vi "Generate Hash Code.vi"(7 "Hash":enum16{"MD5", "FNV-1"}(ring)=enum."FNV-1", 10 "Fingerprint":string, 11 "Product ID":string) -> (2 "Hash":string, 3 "Encrypt":string)   [LabVIEW 2013]
uses:
  <userlib>/_OpenG.lib/md5/md5.llb/MD5 Message Digest (Hexadecimal String)__ogtk.vi
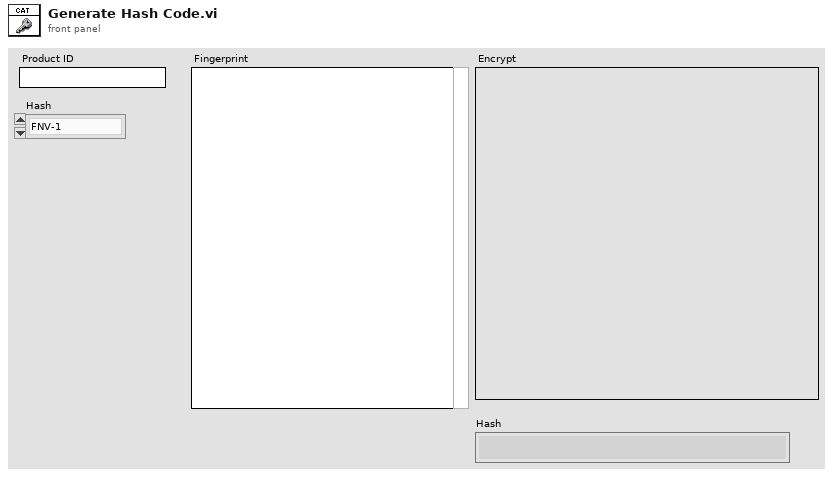
[diagram p1: front panel]
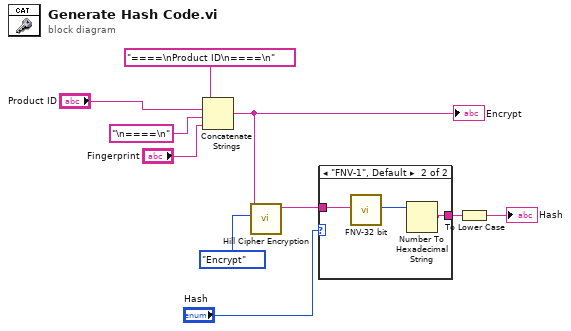
[diagram p0: block diagram]
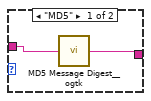
[diagram p2: hidden frame]
diagram:
  n1 = Concatenate Strings("====\nProduct ID\n====\n", "Product ID", "\n====\n" ("string"), "Fingerprint") -> (w10:string)
  "Encrypt" <- w10
  n2 = call <userlib>:"Hill Cipher Encryption.vi"("Operation"=enum16{"Encrypt", "Decrypt", "Decrypt from Hex"}."Encrypt", "Input String"=w10) -> ("Output String"=w4:string)  [unwired: 7 in, 2 out]
  n3 = case shown="\"FNV-1\", Default" "Hash" {
    tunnel: w4 -> [w12 w15]
    tunnel: [w11 w13] -> w2
    frame "MD5" {
      n4 = call-poly <userlib>:"MD5 Message Digest__ogtk.vi"("Message"=w12) -> ("MD5 Message Digest"=w11:string)
    }
    frame "FNV-1", Default {
      n5 = call "FNV-32 bit.vi"("Key"=w15) -> ("32 bit FNV-1 hash"=w14:u32)  [unwired: 18 in]
      n6 = Number To Hexadecimal String(2:w14) -> (0:w13:string)  [unwired: 1 in]
    }
  }
  n7 = To Lower Case(string=w2) -> (all lower case string=→"Hash":string)
